vi "Configure Trigger.vi"(8 "error in":errorcluster, 11 "PXI-5441 Base CFG in":refnum<class "Fgen PXI CFG.lvclass">) -> (0 "error out":errorcluster, 3 "PXI-5441 Base CFG out":refnum<class "Fgen PXI CFG.lvclass">)   [LabVIEW 2023, in "FGEN.lvlib" / "Fgen PXI.lvlib" / "Fgen PXI CFG.lvclass"]
uses:
  Fgen PXI CFG.lvclass
  Fgen PXI CFG.lvclass/Fgen PXI CFG.ctl
  Configuration Base/Configuration Base.lvclass/Configuration Base.ctl
  <instrlib>/niFgen/niFgen.llb/niFgen_ctl Exported Signal Identifiers (Ring).ctl
  <instrlib>/niFgen/niFgen.llb/niFgen_ctl Exported Signal Name Values (Ring).ctl
  <instrlib>/niFgen/niFgen.llb/niFgen_ctl Exported Signal Desination Values (ComboBox).ctl
  7f35fe45-3e00-472d-b8e9-38e85be65bd6.vi
  3014ee4c-903c-46b6-8956-51a497c0a8c9.vi
  fcf7db4a-5ce2-4666-a8dc-47374f3760c0.vi
  ad1c0249-d764-49ee-9182-2bf8b6d34537.vi
  f955f06c-45e7-441c-abc8-c83babd5f264.vi
  <vilib>/JDP Science/JSONtext/Find Item.vi
  <vilib>/JDP Science/JSONtext/Next JSON Value.vi
  <vilib>/JDP Science/JSONtext/String Subset.vi
  <vilib>/JDP Science/JSONtext/Parsing/Advance past next JSON Value (inlined COPY).vi
  <vilib>/JDP Science/JSONtext/Parsing/Advance past whitespace.vi
  <vilib>/JDP Science/JSONtext/Parsing/Advance past String.vi
  <vilib>/JDP Science/JSONtext/Parsing/Advance past Number.vi
  <vilib>/JDP Science/JSONtext/Parsing/Advance past Line Ending.vi
  <vilib>/JDP Science/JSONtext/Parsing/Parse Full Path or Item Name.vi
  <vilib>/JDP Science/JSONtext/Parsing/Advance past Array.vi
  <vilib>/JDP Science/JSONtext/Parsing/Advance past Object.vi
  <vilib>/JDP Science/JSONtext/support/Error Cluster From Code.vi
  <vilib>/JDP Science/JSONtext/Offset/Find Item Locations by Path.vi
  <vilib>/JDP Science/JSONtext/JSON text to Variant.vi
  <vilib>/Utility/error.llb/Error Cluster From Error Code.vi
  <vilib>/JDP Science/JSONtext/LVClass Serializer/JSONtext LVClass Serializer.lvclass
  <vilib>/ErrorRing/Error Ring.xnode
  Configuration Base/Configuration Base.lvclass
  D:/git/HAL/Configuration Base/Configuration Base.lvclass
  D:/git/HAL/Interfaces/IConfigure/IConfigure.lvclass
  D:/git/HAL/Fgen PXI/Fgen PXI CFG/Fgen PXI CFG.lvclass
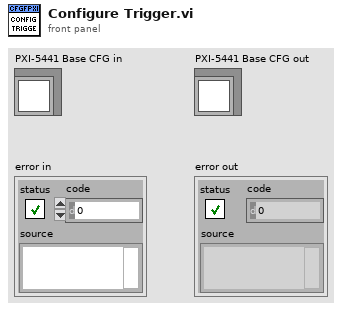
[diagram p1: front panel]
types:
  T1 = typedef "niFgen_ctl Exported Signal Desination Values (ComboBox).ctl" = string
  T2 = typedef "niFgen_ctl Exported Signal Identifiers (Ring).ctl" = string
  T3 = typedef "niFgen_ctl Exported Signal Name Values (Ring).ctl" = u16
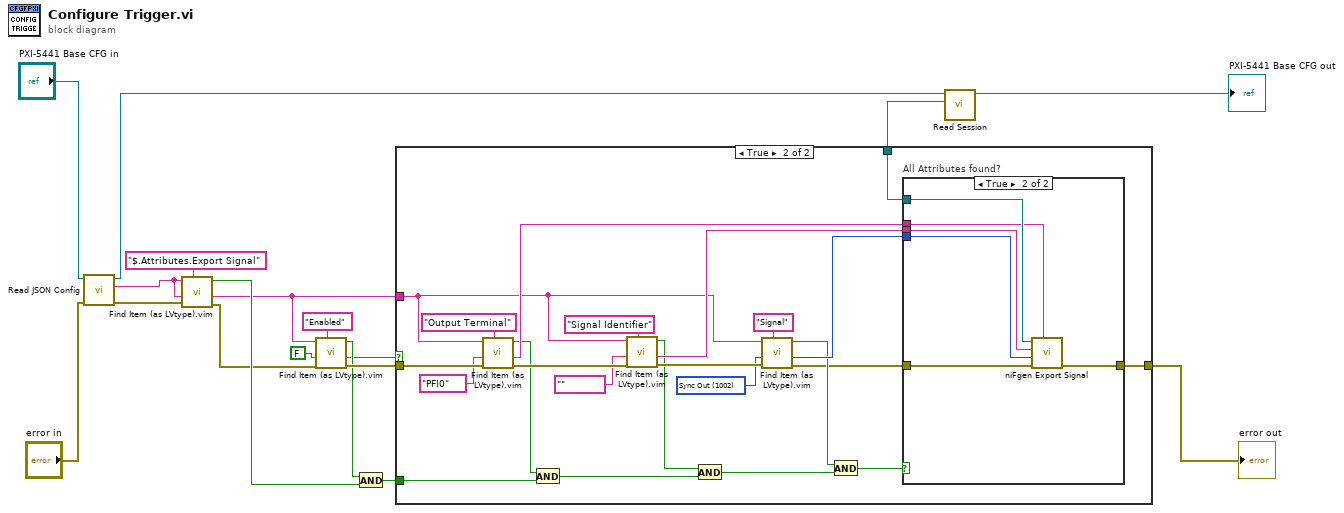
[diagram p0: block diagram]
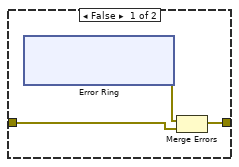
[diagram p3: hidden frame]
diagram:
  n1 = call "Read JSON Config.vi"("error in"="error in", "object in"="PXI-5441 Base CFG in") -> ("error out"=w15:errorcluster, "<JSON>Config"=w1:string, "object out"=w14:refnum<class "Fgen PXI CFG.lvclass">)  [unwired: 7 in]
  n2 = call "Find Item (as LVtype).vim"("$Path or Item Name"="$.Attributes.Export Signal", "error in (no error)"=w15, "Data Type and Default Value"=w1, "JSON"=w1) -> ("error out"=w3:errorcluster, "Data"=w2:string, "Found"=w10:bool)  [unwired: 4 in, 1 out]
  n3 = call "Find Item (as LVtype).vim"("$Path or Item Name"="Enabled", "error in (no error)"=w3, "Data Type and Default Value"=FALSE, "JSON"=w2) -> ("error out"=w9:errorcluster, "Data"=w4:bool, "Found"=w6:bool)  [unwired: 4 in, 1 out]
  n4 = And(x=w6, y=w10) -> (x .and. y?=w7:bool)
  n5 = call "Read Session.vi"("Fgen PXI CFG in"=w14) -> ("Session"=w13:refnum<k15>, "Fgen PXI CFG out"=→"PXI-5441 Base CFG out":refnum<class "Fgen PXI CFG.lvclass">)  [unwired: 8 in, 1 out]
  n6 = case shown="True" w4 {
    tunnel: [w19 w42] -> w11
    tunnel: w9 -> [w19 w33]
    tunnel: w7 -> [_ w32]
    tunnel: w2 -> [_ w26]
    tunnel: w13 -> [_ w25]
    frame False {
    }
    frame True {
      w24 = T3 1002 items=["Sample Clock"=101, "Sample Clock Timebase"=1006, "Reference Clock"=102, "Onboard Reference Clock"=1019, "Start Trigger"=1004, "Script Trigger"=103, "Marker Event"=1001, "Data Marker Event"=108, "Ready For Start Event"=105, "Started Event"=106, "Done Event"=107, "Synchronization Pulse"=1007, "Sync Out"=1002] ("Signal")
      n7 = call "Find Item (as LVtype).vim"("$Path or Item Name"="Output Terminal", "error in (no error)"=w33, "Data Type and Default Value"=T1 "PFI0" ("Output Terminal (do not export)"), "JSON"=w26) -> ("error out"=w40:errorcluster, "Data"=w37:T1, "Found"=w31:bool)  [unwired: 4 in, 1 out]
      n8 = And(x=w31, y=w32) -> (x .and. y?=w29:bool)
      n9 = call "Find Item (as LVtype).vim"("$Path or Item Name"="Signal Identifier", "error in (no error)"=w40, "Data Type and Default Value"=T2 "" ("Signal Identifier (None)"), "JSON"=w26) -> ("error out"=w39:errorcluster, "Data"=w36:T2, "Found"=w30:bool)  [unwired: 4 in, 1 out]
      n10 = And(x=w30, y=w29) -> (x .and. y?=w27:bool)
      n11 = call "Find Item (as LVtype).vim"("$Path or Item Name"="Signal", "error in (no error)"=w39, "Data Type and Default Value"=w24, "JSON"=w26) -> ("error out"=w20:errorcluster, "Data"=w35:T3, "Found"=w28:bool)  [unwired: 4 in, 1 out]
      n12 = And(x=w28, y=w27) -> (x .and. y?=w21:bool)
      n13 = case "All Attributes found?" shown="True" w21 {
        tunnel: w37 -> [_ w54]
        tunnel: w36 -> [_ w53]
        tunnel: w35 -> [_ w52]
        tunnel: [w44 w51] -> w42
        tunnel: w25 -> [_ w55]
        tunnel: w20 -> [w43 w56]
        frame False {
          n14 = xnode "Error Ring"() -> ("error out"=w45:errorcluster)
          n15 = Merge Errors(w45, w43) -> (w44:errorcluster)
        }
        frame True {
          n16 = call <instrlib>:"niFgen Export Signal.vi"("Output Terminal (do not export)"=w54, "error in (no error)"=w56, "Signal"=w52, "Signal Identifier (None)"=w53, "Instrument Handle"=w55) -> ("error out"=w51:errorcluster)  [unwired: 5 in, 1 out]
        }
      }
    }
  }
  "error out" <- w11
